vi "test_VISAInstrument_InitializeSessionWithUnregisteredSessionReserved_RemoteSessionInitialized.vi"(8 "error in":errorcluster) -> (0 "error out":errorcluster, 2 "result":string, 3 "pass":bool)   [LabVIEW 2020, in "MeasurementServerTests.lvlib"]
uses:
  MeasurementServerTests.lvlib
  Runtime/Sessions/VISA Sessions/Plug-In SDK VISA Sessions.lvlib
  Runtime/Sessions/VISA Sessions/Initialize Sessions - 1Sess.vi
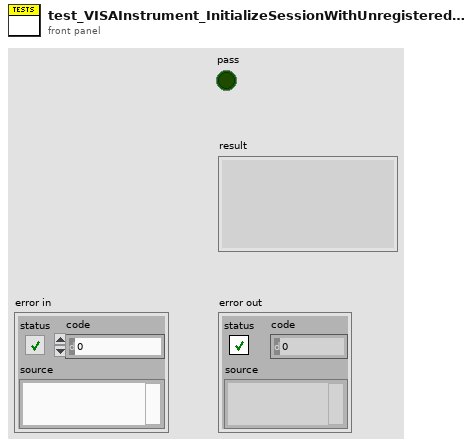
[diagram p1: front panel]
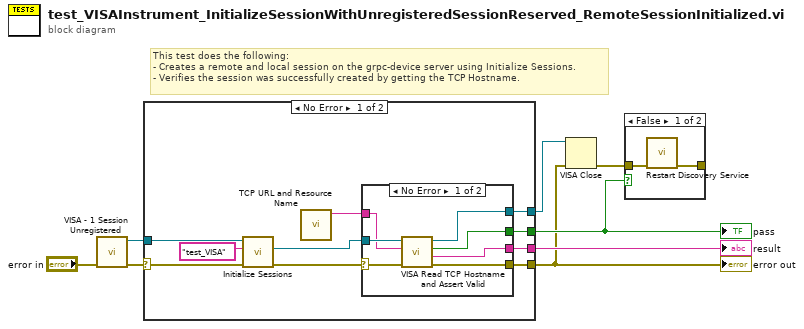
[diagram p0: block diagram]
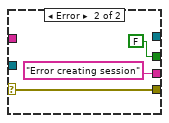
[diagram p2: hidden frame]
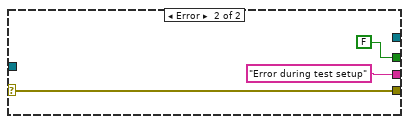
[diagram p3: hidden frame]
diagram:
  # "This test does the following:\n- Creates a remote and local session on the grpc-device server using Initialize Sessions.\n- Verifies the session was successfully created by getting the TCP Hostname."
  n1 = call "VISA - 1 Session Unregistered.vi"("error in"="error in") -> ("error out"=w2:errorcluster, "session reservation out"=w1:refnum<class "Session Reservation.lvclass">)  [unwired: 9 in]
  n2 = case shown="No Error" w2 {
    selector: w2 -> [w13 w29]
    tunnel: [w17 w29] -> w4
    tunnel: [w18 FALSE] -> w5
    tunnel: [w16 "Error during test setup" ("f")] -> w8
    tunnel: [w15 _] -> w7
    tunnel: w1 -> [w12 _]
    frame No Error {
      n3 = call-poly "Initialize Sessions.vi"("error in"=w13, "instrument type id"="test_VISA", "session reservation in"=w12) -> ("error out"=w11:errorcluster, "session"=w14:refnum<visa-resource-name>)  [unwired: 5 in, 2 out]
      n4 = call "TCP URL and Resource Name.vi"() -> ("url"=w9:string)  [unwired: 10 in, 1 out]
      n5 = case shown="No Error" w11 {
        selector: w11 -> [w25 w27]
        tunnel: [w22 FALSE] -> w18
        tunnel: [w20 w27] -> w17
        tunnel: [w21 "Error creating session"] -> w16
        tunnel: w14 -> [w24 _]
        tunnel: [w23 _] -> w15
        tunnel: w9 -> [w19 _]
        frame No Error {
          n6 = call "VISA Read TCP Hostname and Assert Valid.vi"("error in"=w25, "expected hostname"=w19, "visa refnum in"=w24) -> ("error out"=w20:errorcluster, "result"=w21:string, "pass?"=w22:bool, "visa refnum out"=w23:refnum<visa-resource-name>)  [unwired: 5 in]
        }
        frame Error {
        }
      }
    }
    frame Error {
    }
  }
  "error out" <- w4
  "pass" <- w5
  "result" <- w8
  n7 = VISA Close(VISA resource name=w7, error in (no error)=w4) -> (error out=w6:errorcluster)
  n8 = case shown="False" w5 {
    tunnel: w6 -> [w33 _]
    tunnel: [w32 _] -> _
    frame False {
      n9 = call "Restart Discovery Service.vi"("error in"=w33) -> ("error out"=w32:errorcluster)  [unwired: 10 in]
    }
    frame True {
    }
  }
